vi "Acceleration-Operation.vi"(7 "Reset":bool, 9 "迴圈( I )":dbl, 11 "計算設置":cluster{"總位移量":dbl, "最高速":dbl, "加速度":dbl}) -> (0 "完成?":bool[](array[boolean]), 3 "速度":dbl, 4 "三角形?":bool)   [LabVIEW 2019]
panel:
  out "Waveform Chart":dbl(graph)
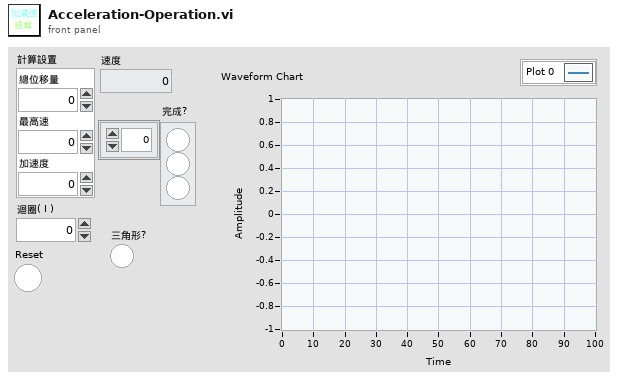
[diagram p1: front panel]
types:
  T1 = cluster{"三角形?":bool, "T1":dbl, "T2":dbl, "T3":dbl, "真實最高速":dbl}
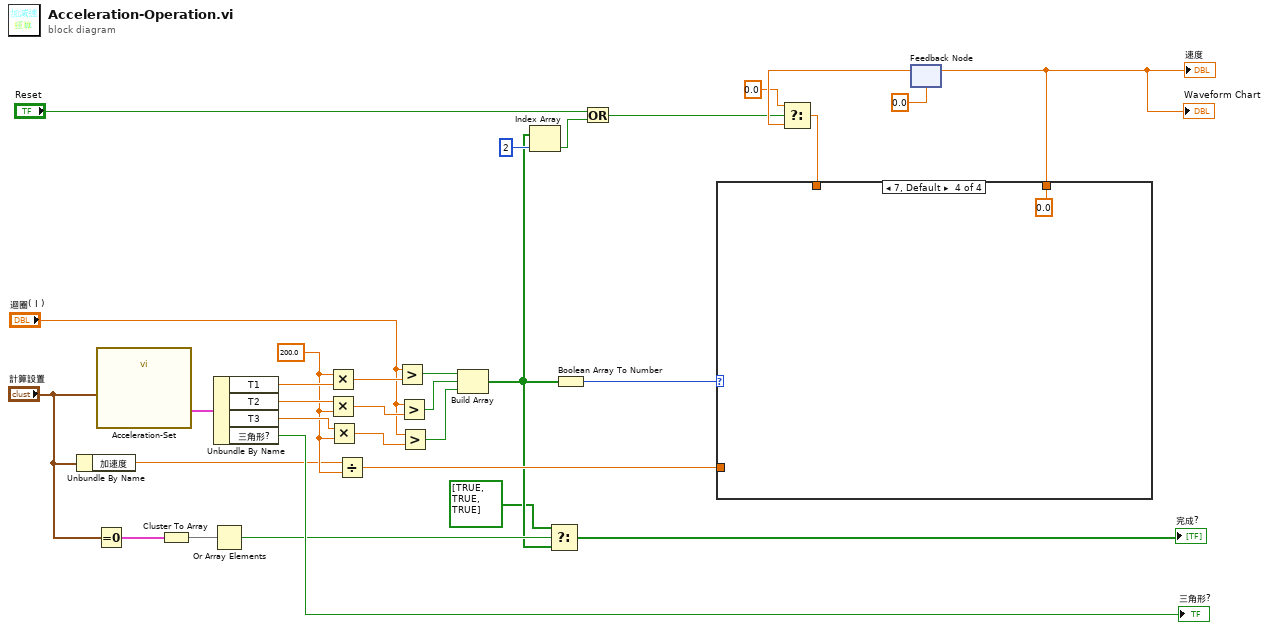
[diagram p0: block diagram]
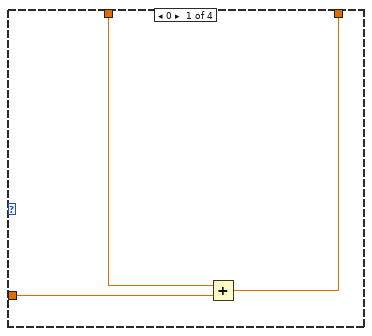
[diagram p2: hidden frame]
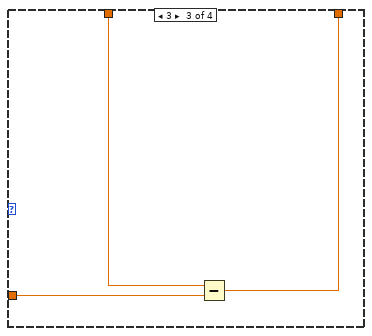
[diagram p4: hidden frame]
diagram:
  w20 = 200.0 ("x")
  n1 = Unbundle By Name("計算設置") -> ("加速度"=w9:dbl)
  n2 = Equal To 0?(x="計算設置") -> (x = 0?=w6:cluster{"總位移量":bool, "最高速":bool, "加速度":bool})
  n3 = call "Acceleration-Set.vi"("計算設置"="計算設置") -> ("輸出結果"=w32:T1)  [unwired: 10 in]
  n4 = Cluster To Array(cluster=w6) -> (array=w5:bool[])
  n5 = Unbundle By Name(w32) -> ("T1"=w30:dbl, "T2"=w31:dbl, "T3"=w29:dbl, "三角形?"=→"三角形?":bool)
  n6 = Or Array Elements(Boolean array=w5) -> (logical OR=w4:bool)
  n7 = Multiply(x=w20, y=w30) -> (x*y=w28:dbl)
  n8 = Multiply(x=w31, y=w20) -> (x*y=w27:dbl)
  n9 = Multiply(x=w29, y=w20) -> (x*y=w26:dbl)
  n10 = Divide(x=w9, y=w20) -> (x/y=w19:dbl)
  n11 = Greater?(x="迴圈( I )", y=w28) -> (0:w24:bool)
  n12 = Greater?(x="迴圈( I )", y=w27) -> (0:w23:bool)
  n13 = Greater?(x="迴圈( I )", y=w26) -> (0:w22:bool)
  n14 = Build Array(w24, w23, w22) -> (w3:bool[])
  n15 = Index Array(array=w3, index=2) -> (element=w13:bool)
  n16 = Select(t=bool[] [TRUE, TRUE, TRUE], s=w4, f=w3) -> (s? t:f=→"完成?":bool[])
  n17 = Boolean Array To Number(Boolean array=w3) -> (number=w21:u32)
  n18 = Or(x="Reset", y=w13) -> (x .or. y?=w15:bool)
  n19 = feedback #1(0.0 ("t")) -> (w17:dbl)
  n20 = Select(t=0.0, s=w15, f=w17) -> (s? t:f=w18:dbl)
  n21 = case shown="7, Default" w21 {
    tunnel: [w35 w36 w39 0.0] -> w10
    tunnel: w18 -> [w34 w36 w38 _]
    tunnel: w19 -> [w33 _ w37 _]
    frame 0 {
      n22 = Add(x=w34, y=w33) -> (x+y=w35:dbl)
    }
    frame 1 {
    }
    frame 3 {
      n23 = Subtract(x=w38, y=w37) -> (x-y=w39:dbl)
    }
    frame 7, Default {
    }
  }
  "速度" <- w10
  "Waveform Chart" <- w10
  n24 = feedback-in #1(w10) -> ()
